vi "בדיקת מפל מתח בין הדקי הממסר תחת עומס bis5.vi"(8 "error":errorcluster, 10 "lines":tag="PXI1Slot8/port0/line1", 11 "Path for Log":path) -> (0 "error IO":errorcluster, 1 "בטוח כן/לא":bool, 2 "מפל מתח בין דקי הממסר תחת עומס":dbl, 3 "תוצאה זמנית":dbl)   [LabVIEW 2015]
uses:
  M9700 Driver/85/vi.lib/M9700 Modbus.llb/CTL Register Address.ctl
  M9700 Driver/86/vi.lib/M9700 Modbus.llb/CTL CMD Register.ctl
  <vilib>/DAQmx/write.llb/DAQmx Write (Digital Bool 1Line 1Point).vi
  <vilib>/Instr/_visa.llb/VISA Configure Serial Port (Instr).vi
  <vilib>/DAQmx/create/channels.llb/DAQmx Create Channel (DO-Digital Output).vi
  <vilib>/DAQmx/miscellaneous.llb/DAQmx Fill In Error Info.vi
panel:
  out "progress":dbl(slide) min=0.0 max=10.0 scale=0.0..10.0
  in  "stop":bool
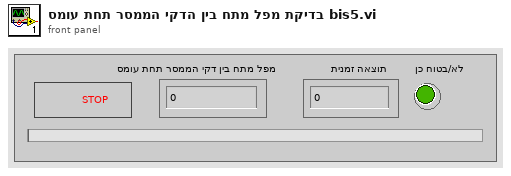
[diagram p1: front panel]
types:
  T1 = enum32{"Invalid", "Standard", "Closed", "Hidden", "Minimized", "Maximized"}
  T2 = typedef "CTL CMD Register.ctl" = u8
  T3 = typedef "CTL Register Address.ctl" = u16
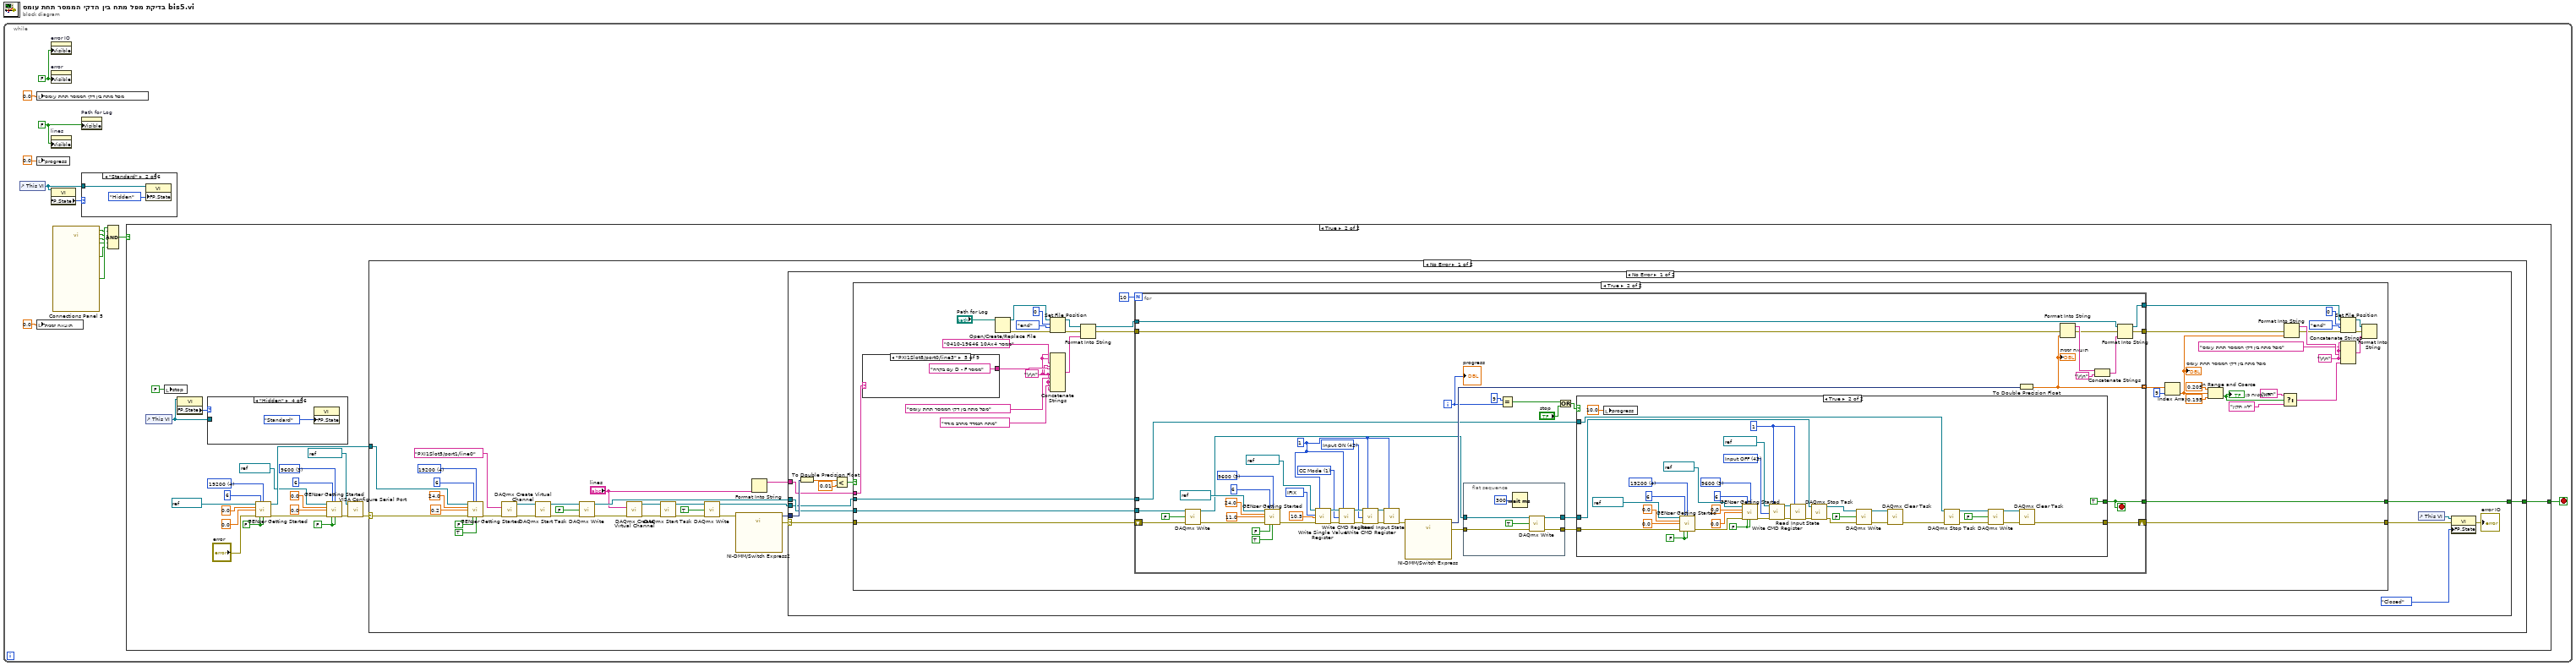
[diagram p0: block diagram]
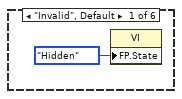
[diagram p2: hidden frame]
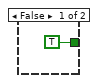
[diagram p7: hidden frame]
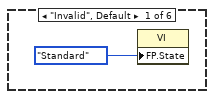
[diagram p8: hidden frame]
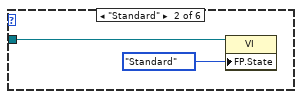
[diagram p9: hidden frame]
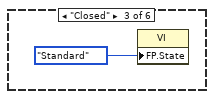
[diagram p10: hidden frame]
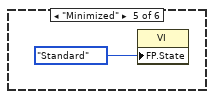
[diagram p11: hidden frame]
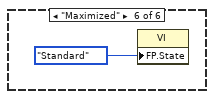
[diagram p12: hidden frame]
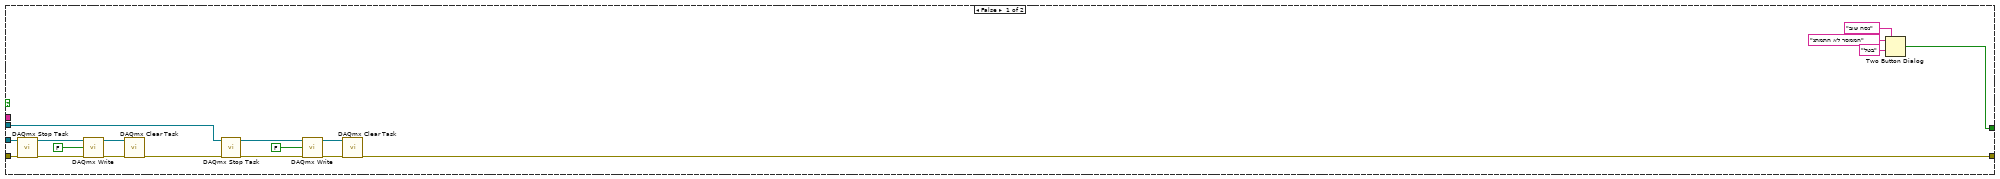
[diagram p13: hidden frame]
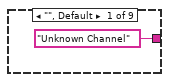
[diagram p14: hidden frame]
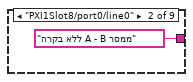
[diagram p15: hidden frame]
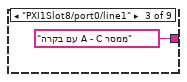
[diagram p16: hidden frame]
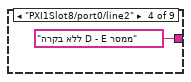
[diagram p17: hidden frame]
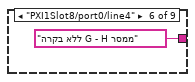
[diagram p18: hidden frame]
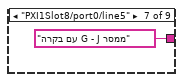
[diagram p19: hidden frame]
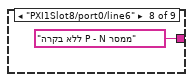
[diagram p20: hidden frame]
diagram:
  n1 = while {
    stop <- w15 stop-if-true
    w3 = FALSE ("Visible")
    w10 = FALSE ("Visible")
    n2 = control-ref of="This VI"() -> (w2:refnum<vi>)
    n3 = local write "מפל מתח בין דקי הממסר תחת עומס"(0.0 ("מפל מתח בין דקי הממסר תחת עומס")) -> ()
    n4 = local write "progress"(0.0 ("progress")) -> ()
    n5 = local write "תוצאה זמנית"(0.0 ("תוצאה זמנית")) -> ()
    n6 = property on="error IO" class="Clust (strict)"("Visible"=w10) -> ()  [unwired: 2 in, 2 out]
    n7 = property on="error" class="Clust (strict)"("Visible"=w10) -> ()  [unwired: 2 in, 2 out]
    n8 = property on="lines" class="DAQmxName"("Visible"=w3) -> ()  [unwired: 2 in, 2 out]
    n9 = property class="VI"(reference=w2) -> ("FP.State"=w1:T1)  [unwired: 1 in, 2 out]
    n10 = call "Connections Panel 5.vi"() -> ("Input Name 10"=w4:bool, "Input Name 6"=w8:bool, "Input Name 7"=w7:bool, "Input Name 8"=w6:bool, "Input Name 9"=w5:bool, "OK"=w9:bool)  [unwired: 13 in, 1 out]
    n11 = property on="Path for Log" class="Path"("Visible"=w3) -> ()  [unwired: 2 in, 2 out]
    n12 = case shown="\"Standard\"" w1 {
      tunnel: w2 -> [_ w17 _ _ _ _]
      frame "Invalid", Default {
        n13 = property class="VI"("FP.State"=T1."Hidden" ("Front Panel Window:State")) -> ()  [unwired: 2 in, 2 out]
      }
      frame "Standard" {
        n14 = property class="VI"(reference=w17, "FP.State"=T1."Hidden" ("Front Panel Window:State")) -> ()  [unwired: 1 in, 2 out]
      }
      frame "Closed" {
      }
      frame "Hidden" {
      }
      frame "Minimized" {
      }
      frame "Maximized" {
      }
    }
    n15 = Compound Arithmetic op=AND(w9, w8, w7, w6, w5, w4) -> (w14:bool)
    n16 = case shown="True" w14 {
      tunnel: [TRUE w28] -> w15
      frame False {
      }
      frame True {
        w24 = FALSE ("Reset (T)")
        w33 = u16 3 items=["1200", "2400", "4800", "9600", "19200"] ("BAUD")
        w23 = FALSE ("Output On (T)")
        w38 = u16 4 items=["1200", "2400", "4800", "9600", "19200"] ("BAUD")
        n17 = control-ref of="This VI"() -> (w20:refnum<vi>)
        n18 = local write "stop"(FALSE ("stop")) -> ()
        n19 = property class="VI"(reference=w20) -> ("FP.State"=w21:T1)  [unwired: 1 in, 2 out]
        n20 = case shown="\"Hidden\"" w21 {
          tunnel: w20 -> [_ w43 _ _ _ _]
          frame "Invalid", Default {
            n21 = property class="VI"("FP.State"=T1."Standard" ("Front Panel Window:State")) -> ()  [unwired: 2 in, 2 out]
          }
          frame "Standard" {
            n22 = property class="VI"(reference=w43, "FP.State"=T1."Standard" ("Front Panel Window:State")) -> ()  [unwired: 1 in, 2 out]
          }
          frame "Closed" {
            n23 = property class="VI"("FP.State"=T1."Standard" ("Front Panel Window:State")) -> ()  [unwired: 2 in, 2 out]
          }
          frame "Hidden" {
            n24 = property class="VI"("FP.State"=T1."Standard" ("Front Panel Window:State")) -> ()  [unwired: 2 in, 2 out]
          }
          frame "Minimized" {
            n25 = property class="VI"("FP.State"=T1."Standard" ("Front Panel Window:State")) -> ()  [unwired: 2 in, 2 out]
          }
          frame "Maximized" {
            n26 = property class="VI"("FP.State"=T1."Standard" ("Front Panel Window:State")) -> ()  [unwired: 2 in, 2 out]
          }
        }
        n27 = call "GENser Getting Started.vi"("VISA"=refnum<visa-resource-name> "COM6", "GEN Addr"=i16 6, "BAUD"=w38, "Voltage Limit"=0.0, "Current Limit"=0.0, "error"="error", "Reset (T)"=w23, "Output On (T)"=w23) -> ("VISA out"=w40:refnum<visa-resource-name>, "error out"=w29:errorcluster)  [unwired: 4 in, 2 out]
        n28 = call "GENser Getting Started.vi"("VISA"=refnum<visa-resource-name> "COM4", "GEN Addr"=i16 6, "BAUD"=w33, "Voltage Limit"=0.0, "Current Limit"=0.0, "error"=w29, "Reset (T)"=w24, "Output On (T)"=w24) -> ("error out"=w26:errorcluster)  [unwired: 4 in, 3 out]
        n29 = call-poly "VISA Configure Serial Port"("VISA resource name"=refnum<visa-resource-name> "COM13", "error in (no error)"=w26) -> ("error out"=w25:errorcluster)  [unwired: 4 in, 9 out]
        n30 = case shown="No Error" w25 {
          selector: w25 -> [w74 _]
          tunnel: w40 -> [w77 _]
          tunnel: [w76 w258] -> w28
          frame No Error {
            w68 = u16 4 items=["1200", "2400", "4800", "9600", "19200"] ("BAUD")
            n31 = call "GENser Getting Started.vi"("VISA"=w77, "GEN Addr"=i16 6, "BAUD"=w68, "Voltage Limit"=24.0, "Current Limit"=0.2, "error"=w74, "Reset (T)"=FALSE, "Output On (T)"=TRUE) -> ("error out"=w62:errorcluster)  [unwired: 4 in, 3 out]
            n32 = call-poly <vilib>:"DAQmx Create Virtual Channel.vi"("lines"=tag "PXI1Slot5/port1/line0", "error in"=w62) -> ("task out"=w58:refnum<k21>, "error out"=w59:errorcluster)  [unwired: 12 in]
            n33 = call <vilib>:"DAQmx Start Task.vi"("task/channels in"=w58, "error in"=w59) -> ("task out"=w56:refnum<k21>, "error out"=w55:errorcluster)  [unwired: 12 in]
            n34 = call-poly <vilib>:"DAQmx Write.vi"("task/channels in"=w56, "data"=FALSE, "error in"=w55) -> ("task out"=w66:refnum<k21>, "error out"=w65:errorcluster)  [unwired: 10 in, 1 out]
            n35 = call-poly <vilib>:"DAQmx Create Virtual Channel.vi"("lines"="lines", "error in"=w65) -> ("task out"=w49:refnum<k21>, "error out"=w50:errorcluster)  [unwired: 12 in]
            n36 = call <vilib>:"DAQmx Start Task.vi"("task/channels in"=w49, "error in"=w50) -> ("task out"=w52:refnum<k21>, "error out"=w51:errorcluster)  [unwired: 12 in]
            n37 = call-poly <vilib>:"DAQmx Write.vi"("task/channels in"=w52, "data"=TRUE, "error in"=w51) -> ("task out"=w64:refnum<k21>, "error out"=w61:errorcluster)  [unwired: 10 in, 1 out]
            n38 = call "NI-DMM/Switch Express2"("error in"=w61) -> ("signals out"=w75:dynamicdata, "error out"=w60:errorcluster)  [unwired: 16 in, 1 out]
            n39 = Format Into String("lines") -> (resulting string=w67:string)  [unwired: 3 in, 1 out]
            n40 = case shown="No Error" w60 {
              selector: w60 -> [w88 _]
              tunnel: [w87 w253] -> w76
              tunnel: w75 -> [w90 _]
              tunnel: w66 -> [w81 _]
              tunnel: w67 -> [w79 _]
              tunnel: w64 -> [w78 _]
              frame No Error {
                n41 = To Double Precision Float(number=w90) -> (double precision float=w86:dbl)
                n42 = Less?(x=w86, y=0.01) -> (x < y?=w89:bool)
                n43 = case shown="True" w89 {
                  tunnel: w88 -> [w98 w112]
                  tunnel: [w91 w150] -> w87
                  tunnel: [w95 w144] -> w82
                  tunnel: w81 -> [w97 w145]
                  tunnel: w79 -> [_ w114]
                  tunnel: w78 -> [w96 w113]
                  frame False {
                    n44 = call <vilib>:"DAQmx Stop Task.vi"("task/channels in"=w97, "error in"=w98) -> ("task out"=w109:refnum<k21>, "error out"=w107:errorcluster)  [unwired: 12 in]
                    n45 = call-poly <vilib>:"DAQmx Write.vi"("task/channels in"=w109, "data"=FALSE, "error in"=w107) -> ("task out"=w106:refnum<k21>, "error out"=w105:errorcluster)  [unwired: 10 in, 1 out]
                    n46 = call <vilib>:"DAQmx Clear Task.vi"("task in"=w106, "error in"=w105) -> ("error out"=w99:errorcluster)  [unwired: 13 in]
                    n47 = call <vilib>:"DAQmx Stop Task.vi"("task/channels in"=w96, "error in"=w99) -> ("task out"=w104:refnum<k21>, "error out"=w102:errorcluster)  [unwired: 12 in]
                    n48 = call-poly <vilib>:"DAQmx Write.vi"("task/channels in"=w104, "data"=FALSE, "error in"=w102) -> ("task out"=w101:refnum<k21>, "error out"=w100:errorcluster)  [unwired: 10 in, 1 out]
                    n49 = call <vilib>:"DAQmx Clear Task.vi"("task in"=w101, "error in"=w100) -> ("error out"=w95:errorcluster)  [unwired: 13 in]
                    n50 = Two Button Dialog(message="הממסר לא התמתג", 1:"נסה שוב" ("F button name (\"Cancel\")"), 2:"בטל" ("T button name (\"OK\")")) -> (T button?=w91:bool)
                  }
                  frame True {
                    w131 = "\r\n"
                    w110 = "\r\n"
                    n51 = case shown="\"PXI1Slot8/port0/line3\"" w114 {
                      tunnel: ["Unknown Channel" "ללא בקרה A - B ממסר" "עם בקרה A - C ממסר" "ללא בקרה D - E ממסר" "עם בקרה D - F ממסר" "ללא בקרה G - H ממסר" "עם בקרה G - J ממסר" "ללא בקרה P - N ממסר" "עם בקרה P - L ממסר"] -> w111
                      frame "", Default {
                      }
                      frame "PXI1Slot8/port0/line0" {
                      }
                      frame "PXI1Slot8/port0/line1" {
                      }
                      frame "PXI1Slot8/port0/line2" {
                      }
                      frame "PXI1Slot8/port0/line3" {
                      }
                      frame "PXI1Slot8/port0/line4" {
                      }
                      frame "PXI1Slot8/port0/line5" {
                      }
                      frame "PXI1Slot8/port0/line6" {
                      }
                      frame "PXI1Slot8/port0/line7" {
                      }
                    }
                    n52 = Open/Create/Replace File(file path (use dialog)="Path for Log") -> (refnum out=w141:refnum<file>, error out=w140:errorcluster)  [unwired: 5 in, 1 out]
                    n53 = Set File Position(offset (in bytes) (0)=i64 0, refnum=w141, from (0:start)=enum16{"start", "end", "current"}."end", error in=w140) -> (refnum out=w137:refnum<file>, error out=w134:errorcluster)
                    n54 = Concatenate Strings(w110, w110, "0410-19646 10Ax4 ממסר", w110, w111, w110, "מפל מתח בין דקי הממסר תחת עומס", w110, "מתח הנמדד מהרב מודד", w110) -> (w139:string)
                    n55 = Format Into String(initial string=w137, error in=w134, w139) -> (resulting string=w132:refnum<file>, error out=w133:errorcluster)  [unwired: 1 in]
                    n56 = for {
                      N: 10 -> [_]
                      tunnel: [w183] -> w150
                      shift-right: [w180] -> w144
                      shift-left: w112 -> [w175]
                      tunnel: [w161] -> w149 mode=indexing
                      tunnel: w145 -> [w176]
                      tunnel: w133 -> [w165]
                      tunnel: w132 -> [w167]
                      tunnel: [w164] -> w125
                      tunnel: [w163] -> w116
                      tunnel: w113 -> [w162]
                      i -> [w179]
                      stop <- w183 stop-if-true
                      w191 = T2 42 items=["CC Mode"=1, "CV Mode"=2, "CW Mode"=3, "CR Mode"=4, "Short Mode"=26, "Set SysPara"=41, "Input ON"=42, "Input OFF"=43] ("CMD Register Value")
                      w194 = u8 1 ("Load Address")
                      w198 = T2 1 items=["CC Mode"=1, "CV Mode"=2, "CW Mode"=3, "CR Mode"=4, "Short Mode"=26, "Set SysPara"=41, "Input ON"=42, "Input OFF"=43] ("CMD Register Value")
                      w201 = T3 2561 items=["REMOTE"=1283, "ISTATE"=1296, "CMD"=2560, "IFIX"=2561, "UFIX"=2563, "PFIX"=2565, "RFIX"=2567, "IMAX"=2612, "UMAX"=2614, "PMAX"=2616, "U"=2816, "I"=2818, "MODEL"=2822, "EDITION"=2823] ("Register Address")
                      w206 = u16 3 items=["1200", "2400", "4800", "9600", "19200"] ("BAUD")
                      n57 = call-poly <vilib>:"DAQmx Write.vi"("task/channels in"=w176, "data"=FALSE, "error in"=w175) -> ("task out"=w174:refnum<k21>, "error out"=w173:errorcluster)  [unwired: 10 in, 1 out]
                      n58 = call "GENser Getting Started.vi"("VISA"=refnum<visa-resource-name> "COM4", "GEN Addr"=i16 6, "BAUD"=w206, "Voltage Limit"=24.0, "Current Limit"=11.0, "error"=w173, "Reset (T)"=FALSE, "Output On (T)"=TRUE) -> ("error out"=w196:errorcluster)  [unwired: 4 in, 3 out]
                      n59 = call "Write Single Value Register.vi"("VISA resource name"=refnum<visa-resource-name> "COM13", "Starting Address(HEX)"=w201, "Register Single Value"=sgl 10.5, "error in"=w196, "Load Address"=w194) -> ("VISA resource name out"=w200:refnum<visa-resource-name>, "error out"=w199:errorcluster)  [unwired: 13 out]
                      n60 = call "Write CMD Register.vi"("VISA resource name"=w200, "CMD Value"=w198, "error in"=w199, "Load Address"=w194) -> ("VISA resource name out"=w195:refnum<visa-resource-name>, "error out"=w192:errorcluster)  [unwired: 14 out]
                      n61 = call "Write CMD Register.vi"("VISA resource name"=w195, "CMD Value"=w191, "error in"=w192, "Load Address"=w194) -> ("VISA resource name out"=w193:refnum<visa-resource-name>, "error out"=w190:errorcluster)  [unwired: 14 out]
                      n62 = call "Read Input State.vi"("VISA resource name"=w193, "error in"=w190, "Load Address"=w194) -> ("error out"=w189:errorcluster)  [unwired: 16 out]
                      n63 = call "NI-DMM/Switch Express"("error in"=w189) -> ("signals out"=w188:dynamicdata, "error out"=w177:errorcluster)  [unwired: 16 in, 1 out]
                      n64 = flat-sequence {
                        tunnel: [w213] -> w178
                        tunnel: w177 -> [w212]
                        tunnel: w174 -> [w210]
                        tunnel: [w209] -> w171
                        frame #0 {
                          n65 = Wait (ms)(milliseconds to wait=u32 300) -> ()  [unwired: 1 out]
                          n66 = call-poly <vilib>:"DAQmx Write.vi"("task/channels in"=w210, "data"=TRUE, "error in"=w212) -> ("task out"=w209:refnum<k21>, "error out"=w213:errorcluster)  [unwired: 10 in, 1 out]
                        }
                      }
                      n67 = Equal?(x=9, y=w179) -> (x = y?=w185:bool)
                      n68 = Or(x=w185, y="stop") -> (x .or. y?=w186:bool)
                      n69 = case shown="True" w186 {
                        tunnel: [FALSE TRUE] -> w183
                        tunnel: w178 -> [w214 w241]
                        tunnel: [w214 w218] -> w180
                        tunnel: w171 -> [_ w224]
                        tunnel: w162 -> [_ w216]
                        frame False {
                        }
                        frame True {
                          w232 = u8 1 ("Load Address")
                          w235 = T2 43 items=["CC Mode"=1, "CV Mode"=2, "CW Mode"=3, "CR Mode"=4, "Short Mode"=26, "Set SysPara"=41, "Input ON"=42, "Input OFF"=43] ("CMD Register Value")
                          w239 = FALSE ("Reset (T)")
                          w245 = u16 3 items=["1200", "2400", "4800", "9600", "19200"] ("BAUD")
                          w238 = FALSE ("Reset (T)")
                          w248 = u16 4 items=["1200", "2400", "4800", "9600", "19200"] ("BAUD")
                          n70 = local write "progress"(10.0 ("progress")) -> ()
                          n71 = call "GENser Getting Started.vi"("VISA"=refnum<visa-resource-name> "COM6", "GEN Addr"=i16 6, "BAUD"=w248, "Voltage Limit"=0.0, "Current Limit"=0.0, "error"=w241, "Reset (T)"=w238, "Output On (T)"=w238) -> ("error out"=w240:errorcluster)  [unwired: 4 in, 3 out]
                          n72 = call "GENser Getting Started.vi"("VISA"=refnum<visa-resource-name> "COM4", "GEN Addr"=i16 6, "BAUD"=w245, "Voltage Limit"=0.0, "Current Limit"=0.0, "error"=w240, "Reset (T)"=w239, "Output On (T)"=w239) -> ("error out"=w237:errorcluster)  [unwired: 4 in, 3 out]
                          n73 = call "Write CMD Register.vi"("VISA resource name"=refnum<visa-resource-name> "COM13", "CMD Value"=w235, "error in"=w237, "Load Address"=w232) -> ("VISA resource name out"=w233:refnum<visa-resource-name>, "error out"=w236:errorcluster)  [unwired: 14 out]
                          n74 = call "Read Input State.vi"("VISA resource name"=w233, "error in"=w236, "Load Address"=w232) -> ("error out"=w225:errorcluster)  [unwired: 16 out]
                          n75 = call <vilib>:"DAQmx Stop Task.vi"("task/channels in"=w224, "error in"=w225) -> ("task out"=w230:refnum<k21>, "error out"=w228:errorcluster)  [unwired: 12 in]
                          n76 = call-poly <vilib>:"DAQmx Write.vi"("task/channels in"=w230, "data"=FALSE, "error in"=w228) -> ("task out"=w227:refnum<k21>, "error out"=w226:errorcluster)  [unwired: 10 in, 1 out]
                          n77 = call <vilib>:"DAQmx Clear Task.vi"("task in"=w227, "error in"=w226) -> ("error out"=w217:errorcluster)  [unwired: 13 in]
                          n78 = call <vilib>:"DAQmx Stop Task.vi"("task/channels in"=w216, "error in"=w217) -> ("task out"=w223:refnum<k21>, "error out"=w221:errorcluster)  [unwired: 12 in]
                          n79 = call-poly <vilib>:"DAQmx Write.vi"("task/channels in"=w223, "data"=FALSE, "error in"=w221) -> ("task out"=w220:refnum<k21>, "error out"=w219:errorcluster)  [unwired: 10 in, 1 out]
                          n80 = call <vilib>:"DAQmx Clear Task.vi"("task in"=w220, "error in"=w219) -> ("error out"=w218:errorcluster)  [unwired: 13 in]
                        }
                      }
                      n81 = To Double Precision Float(number=w188) -> (double precision float=w161:dbl)
                      "תוצאה זמנית" <- w161
                      n82 = Format Into String(error in=w165, w161) -> (resulting string=w169:string, error out=w166:errorcluster)  [unwired: 2 in]
                      n83 = Concatenate Strings(w169, "\r\n") -> (w168:string)
                      n84 = Format Into String(initial string=w167, error in=w166, w168) -> (resulting string=w164:refnum<file>, error out=w163:errorcluster)  [unwired: 1 in]
                      "progress" <- w179
                    }
                    n85 = Index Array(array=w149, index=9) -> (element=w124:dbl)
                    "מפל מתח בין דקי הממסר תחת עומס" <- w124
                    n86 = In Range and Coerce(upper limit=0.205, x=w124, lower limit=0.195) -> (In Range?=w119:bool)  [unwired: 1 out]
                    "בטוח כן/לא" <- w119
                    n87 = Select(t="תקין", s=w119, f="לא תקין") -> (s? t:f=w118:string)
                    n88 = Format Into String(error in=w116, w124) -> (resulting string=w123:string, error out=w117:errorcluster)  [unwired: 2 in]
                    n89 = Set File Position(offset (in bytes) (0)=i64 0, refnum=w125, from (0:start)=enum16{"start", "end", "current"}."end", error in=w117) -> (refnum out=w128:refnum<file>, error out=w127:errorcluster)
                    n90 = Concatenate Strings(w131, "מפל מתח בין דקי הממסר תחת עומס" ("string"), w131, w123, w131, w118) -> (w126:string)
                    n91 = Format Into String(initial string=w128, error in=w127, w126) -> ()  [unwired: 1 in, 2 out]
                  }
                }
                n92 = control-ref of="This VI"() -> (w84:refnum<vi>)
                n93 = property class="VI"(reference=w84, error in=w82, "FP.State"=T1."Closed" ("Front Panel Window:State")) -> (error out=→"error IO":errorcluster)  [unwired: 1 out]
              }
              frame Error {
                n94 = Two Button Dialog(message="בעיית דגימת נתונים ע\"י הכרטיס רב מודד", 1:"ביטול" ("F button name (\"Cancel\")"), 2:"נסה שוב" ("T button name (\"OK\")")) -> (T button?=w254:bool)
                n95 = Not(x=w254) -> (.not. x?=w253:bool)
              }
            }
          }
          frame Error {
            n96 = Two Button Dialog(message="בעיית תקשורת עם ספק קוח", 1:"ביטול" ("F button name (\"Cancel\")"), 2:"נסה שוב" ("T button name (\"OK\")")) -> (T button?=w259:bool)
            n97 = Not(x=w259) -> (.not. x?=w258:bool)
          }
        }
      }
    }
  }
